vi "GEOM_BinRemainders.vi"(6 "bin factor":i32, 7 "bin?":bool, 9 "remaining data":i32, 10 "remaining modif":i32) -> (1 "remaining remainder":i32, 2 "out value":i32)   [LabVIEW 2016]
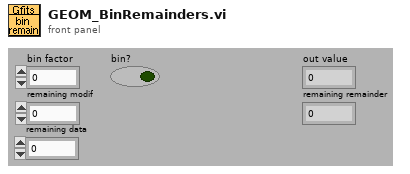
[diagram p1: front panel]
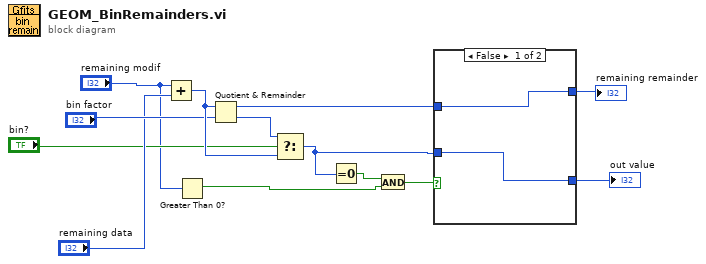
[diagram p0: block diagram]
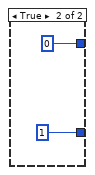
[diagram p2: hidden frame]
diagram:
  n1 = Add(x="remaining modif", y="remaining data") -> (x+y=w12:i32)
  n2 = Greater Than 0?(x="remaining modif") -> (x > 0?=w6:bool)
  n3 = Quotient & Remainder(x=w12, y="bin factor") -> (x-y*floor(x/y)=w1:i32, floor(x/y)=w13:i32)
  n4 = Select(t=w13, s="bin?", f=w12) -> (s? t:f=w2:i32)
  n5 = Equal To 0?(x=w2) -> (x = 0?=w7:bool)
  n6 = And(x=w7, y=w6) -> (x .and. y?=w5:bool)
  n7 = case shown="False" w5 {
    tunnel: [w15 1] -> w4
    tunnel: [w14 0] -> w3
    tunnel: w2 -> [w15 _]
    tunnel: w1 -> [w14 _]
    frame False {
    }
    frame True {
    }
  }
  "remaining remainder" <- w3
  "out value" <- w4
